vi "Move XZ Raster  + Scan.vi"(0 "Reference In":refnum<class "_Controller.lvclass">, 1 "VISA resource name":refnum<visa-resource-name>, 2 "X Number of Steps":string="0", 3 "Z Number of Steps":string="0", 4 "Source (0: Channel 1)":u16(ring) items=["Channel 1", "Channel 2", "Channel 3", "Channel 4", "Memory 1", "Memory 2", "Memory 3", "Memory 4", "Function 1", "Function 2", "Function 3", "Function 4", "Function 5", "Function 6", "Function 7", "Function 8"], 5 "Error In":errorcluster, 8 "C-Scan Build Up Quantity":T1(radio), 9 "Initial X Direction":bool=TRUE, 11 "Initial Z Direction":bool=TRUE) -> (14 "Reference Out":refnum<class "_Controller.lvclass">, 16 "C-Scan":dbl[][](array[numeric]), 17 "A-Scan (for C-Scan)":waveform(dbl)[](graph), 19 "Error Out":errorcluster)   [LabVIEW 2020]
doc: "Bi-axial raster scan logic for the XZ plane. Performs the uni-axial raster scan logic in the X direction then moves along 1 scanning point in the Z dirction. This is the looped to cover the entire area.\n\nArgs:\n\nReference In: Incoming communication (reference) between LabView and the scanning rig controller\nX Number of Steps: Total number of steps to move along that axis\nZ Number of Steps: Total number of steps to move along that axis\nInitial X Direction: Initial X direction for the scan\nInitial Z Direction: Initial Z direction for the scan\nError In: Checks for any errors with the incoming communication (reference)\n\nReturns:\n\nReference Out: Output communnication (reference) between LabView and controller\nError Out: Checks for any error with output communication (reference)"
uses:
  <instrlib>/Arcus Ethernet Driver 1.0.0/ArcusEthernetComm/classes/Controller/_Controller.lvclass
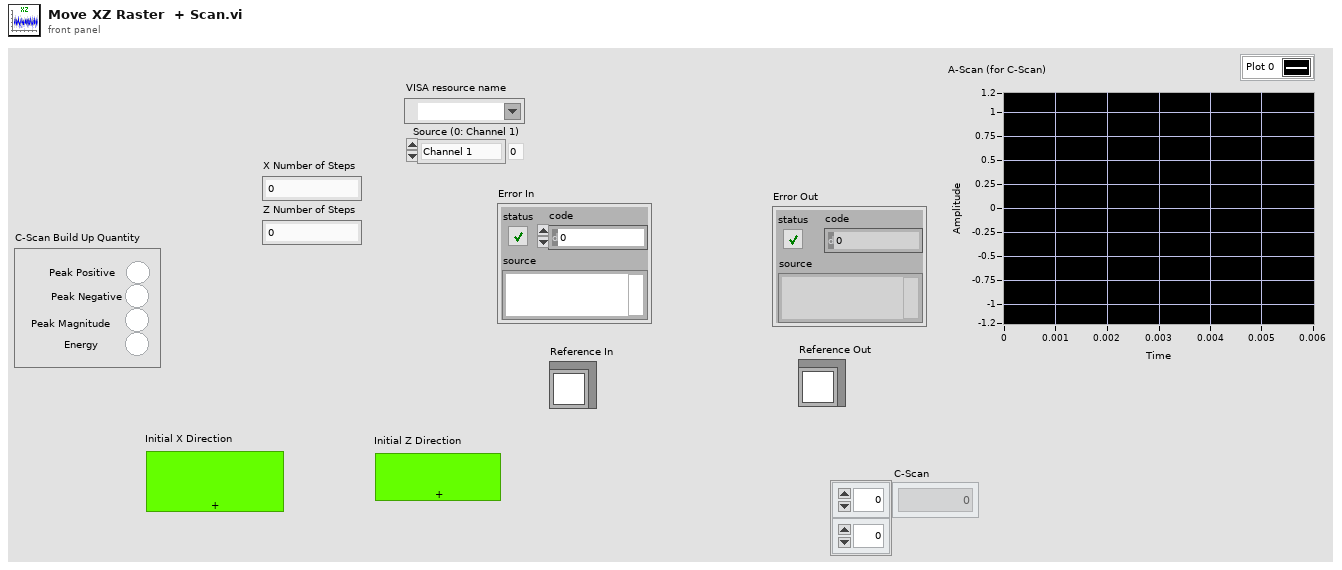
[diagram p1: front panel]
types:
  T1 = enum32{"No Selection", "Peak Positive", "Peak Negative", "Peak Magnitude", "Energy"}
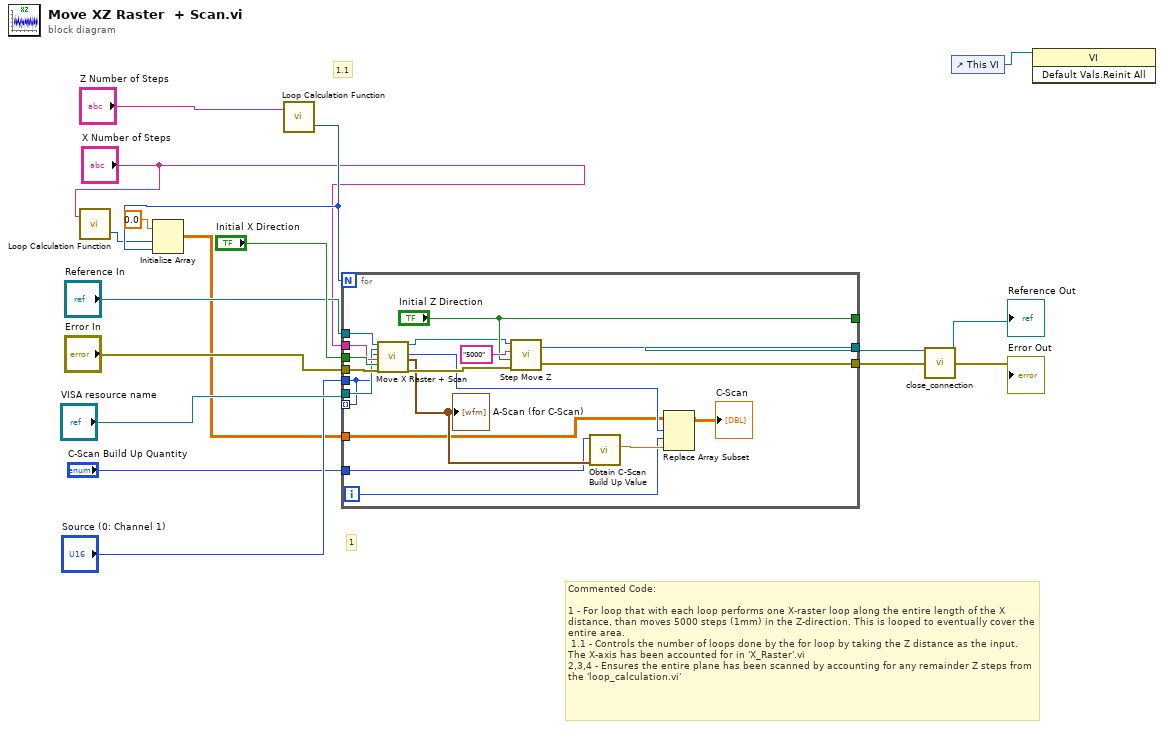
[diagram p0: block diagram]
diagram:
  # "Commented Code:\n\n1 - For loop that with each loop performs one X-raster loop along the entire length of the X distance, than moves 5000 steps (1mm) in the Z-direction. This is looped to eventually cover the entire area.\n 1.1 - Controls the number of loops done by the for loop by taking the Z distance as the input. The X-axis has been accounted for in 'X_Raster'.vi\n2,3,4 - Ensures the entire plane has been scanned by accounting for any remainder Z steps from the 'loop_calculation.vi'"
  # "1.1"
  # "1"
  n1 = call "Loop Calculation Function.vi"("Number of Steps"="X Number of Steps") -> ("No. of Scan Points"=w3:i32)  [unwired: 1 in, 1 out]
  n2 = call "Loop Calculation Function.vi"("Number of Steps"="Z Number of Steps") -> ("No. of Scan Points"=w4:i32)  [unwired: 1 in, 1 out]
  n3 = Initialize Array(0.0 ("element"), w3, w4) -> (w5:dbl[][])
  n4 = for {
    N: w4 -> [_]
    tunnel: "X Number of Steps" -> [w34]
    tunnel: "Initial X Direction" -> [w35]
    tunnel: ["Initial Z Direction"] -> _
    tunnel: [w31] -> w10
    tunnel: [w30] -> w9
    tunnel: "Reference In" -> [w28]
    tunnel: "Error In" -> [w27]
    tunnel: "VISA resource name" -> [w26]
    tunnel: [w25] -> _ mode=indexing
    tunnel: "Source (0: Channel 1)" -> [w25]
    tunnel: w5 -> [w20]
    tunnel: "C-Scan Build Up Quantity" -> [w18]
    i -> [w22]
    n5 = call "Move X Raster + Scan.vi"("Reference In"=w28, "VISA resource name (Osc. Model)"=w26, "Source (0: Channel 1)"=w25, "X Number of Steps"=w34, "Initial Direction"=w35, "Error In"=w27) -> ("Reference Out"=w32:refnum<class "_Controller.lvclass">, "For Loop Count"=w21:i32, "A-Scan"=w23:waveform(dbl)[], "Error Out"=w29:errorcluster)  [unwired: 10 in]
    "A-Scan (for C-Scan)" <- w23
    n6 = call "Step Move Z.vi"("Error In"=w29, "Direction"="Initial Z Direction", "No. of Z Steps"="5000" ("Y Steps"), "Reference In"=w32) -> ("Error Out"=w30:errorcluster, "Reference Out"=w31:refnum<class "_Controller.lvclass">)
    n7 = call "Obtain C-Scan Build Up Value.vi"("A-Scans"=w23, "C-Scan Build Up Quantity"=w18) -> ("Desired Value for C-Scan"=w24:dbl)  [unwired: 9 in]
    n8 = Replace Array Subset(array=w20, new element=w24, index (row)=w21, index (col)=w22) -> (→"C-Scan":dbl[][])
  }
  n9 = call <instrlib>:"close_connection.vi"("reference (in)"=w10, "error in (no error)"=w9) -> ("reference (out)"=→"Reference Out":refnum<class "_Controller.lvclass">, "error out"=→"Error Out":errorcluster)  [unwired: 16 in]
  n10 = control-ref of="This VI"() -> (w12:refnum<vi>)
  n11 = invoke class="VI" method="Default Vals.Reinit All"(reference=w12) -> ()  [unwired: 2 in, 3 out]
